vi "Bundle.vi"(8 "error in (no error)":errorcluster, 10 "New File Path":path, 11 "Open File Msg in":refnum<class "Open File Msg.lvclass">) -> (0 "error out":errorcluster, 3 "Open File Msg out":refnum<class "Open File Msg.lvclass">)   [LabVIEW 2020, in "File Writer.lvlib" / "Open File Msg.lvclass"]
doc: "Write the 'New FIle Path' to the class."
uses:
  Open File Msg.lvclass
  Open File Msg.lvclass/Open File Msg.ctl
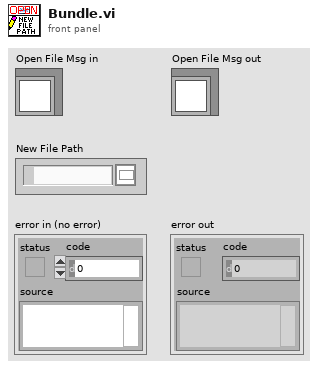
[diagram p1: front panel]
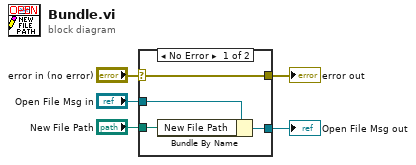
[diagram p0: block diagram]
diagram:
  n1 = case shown="No Error" "error in (no error)" {
    selector: "error in (no error)" -> [w9 w10]
    tunnel: [w9 w10] -> w4
    tunnel: [w7 w11] -> w2
    tunnel: "Open File Msg in" -> [w8 w11]
    tunnel: "New File Path" -> [w6 _]
    frame No Error {
      n2 = Bundle By Name(cluster=w8, "New File Path"=w6) -> (w7:refnum<class "Open File Msg.lvclass">)
    }
    frame Error {
    }
  }
  "error out" <- w4
  "Open File Msg out" <- w2
